vi "Log Datei schreiben.vi"(7 "An Datei Anhängen?":bool, 8 "error in (no error)":errorcluster caption="Fehler (Eingang, kein Fehler)", 9 "Array":string[](array[string]), 10 "Dateipfad":path) -> (0 "error out":errorcluster caption="Fehler (Ausgang)")   [LabVIEW 2020, in "allgemeine Sub-VIs.lvlib"]
uses:
  allgemeine Sub-VIs.lvlib
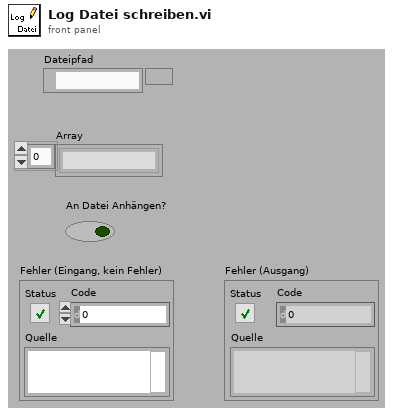
[diagram p1: front panel]
types:
  T1 = enum16{"open", "replace", "create", "open or create", "replace or create", "replace or create with confirmation"}
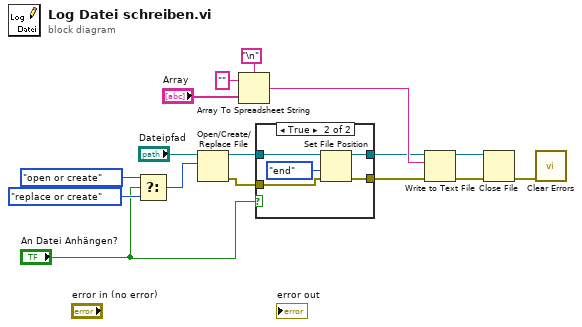
[diagram p0: block diagram]
diagram:
  n1 = Select(t=T1."open or create" ("Operation (0:Öffnen)"), s="An Datei Anhängen?", f=T1."replace or create" ("Operation (0:Öffnen)")) -> (s? t:f=w6:T1)
  n2 = Open/Create/Replace File(file path (use dialog)="Dateipfad", operation (0:open)=w6) -> (refnum out=w5:refnum<file>, error out=w3:errorcluster)  [unwired: 4 in, 1 out]
  n3 = Array To Spreadsheet String(delimiter (Tab)="\n", array="Array", 3:"" ("Format-String")) -> (spreadsheet string=w9:string)
  n4 = case shown="True" "An Datei Anhängen?" {
    tunnel: w5 -> [w18 w22]
    tunnel: [w18 w21] -> w4
    tunnel: w3 -> [w17 w20]
    tunnel: [w17 w19] -> w2
    frame False {
    }
    frame True {
      n5 = Set File Position(refnum=w22, from (0:start)=enum16{"start", "end", "current"}."end" ("Von (0:Start)"), error in=w20) -> (refnum out=w21:refnum<file>, error out=w19:errorcluster)  [unwired: 1 in]
    }
  }
  n6 = Write to Text File(file (use dialog)=w4, text=w9, error in=w2) -> (refnum out=w11:refnum<file>, error out=w10:errorcluster)  [unwired: 1 in, 1 out]
  n7 = Close File(refnum=w11, error in=w10) -> (error out=w15:errorcluster)  [unwired: 1 out]
  n8 = call <vilib>:"Clear Errors.vi"("error in (no error)"=w15) -> ()  [unwired: 5 in, 2 out]
